vi "Create Server.vi"(5 "Server Key File (.key)":path, 7 "Server Certificate File (.crt)":path, 8 "error in (no error)":errorcluster, 11 "Server Address":string) -> (0 "error out":errorcluster, 3 "OOP Server out":refnum<class "Template Server.lvclass">)   [LabVIEW 2019, in "Template Server.lvlib" / "Template Server.lvclass"]
uses:
  Template Server.lvclass
  Template Server.lvclass/Template Server.ctl
  gRPC interface/gprc-lvsupport.lvlib
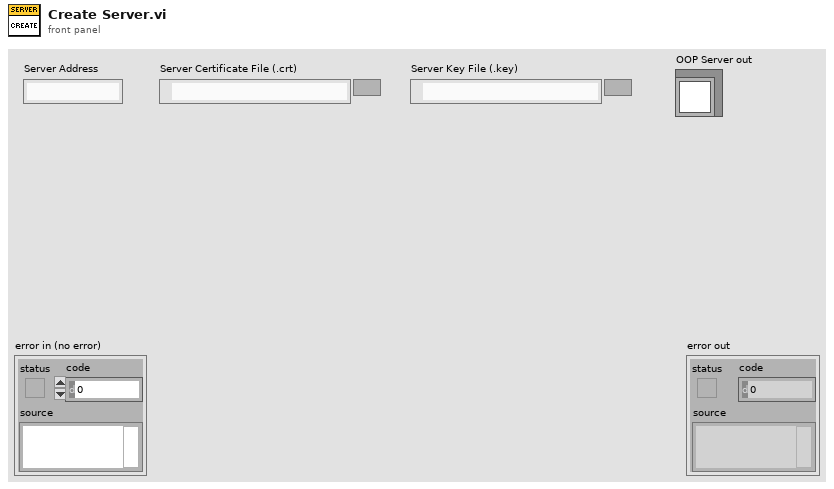
[diagram p1: front panel]
types:
  T1 = typedef "gprc-lvsupport.lvlib/grpcId.ctl" = u64
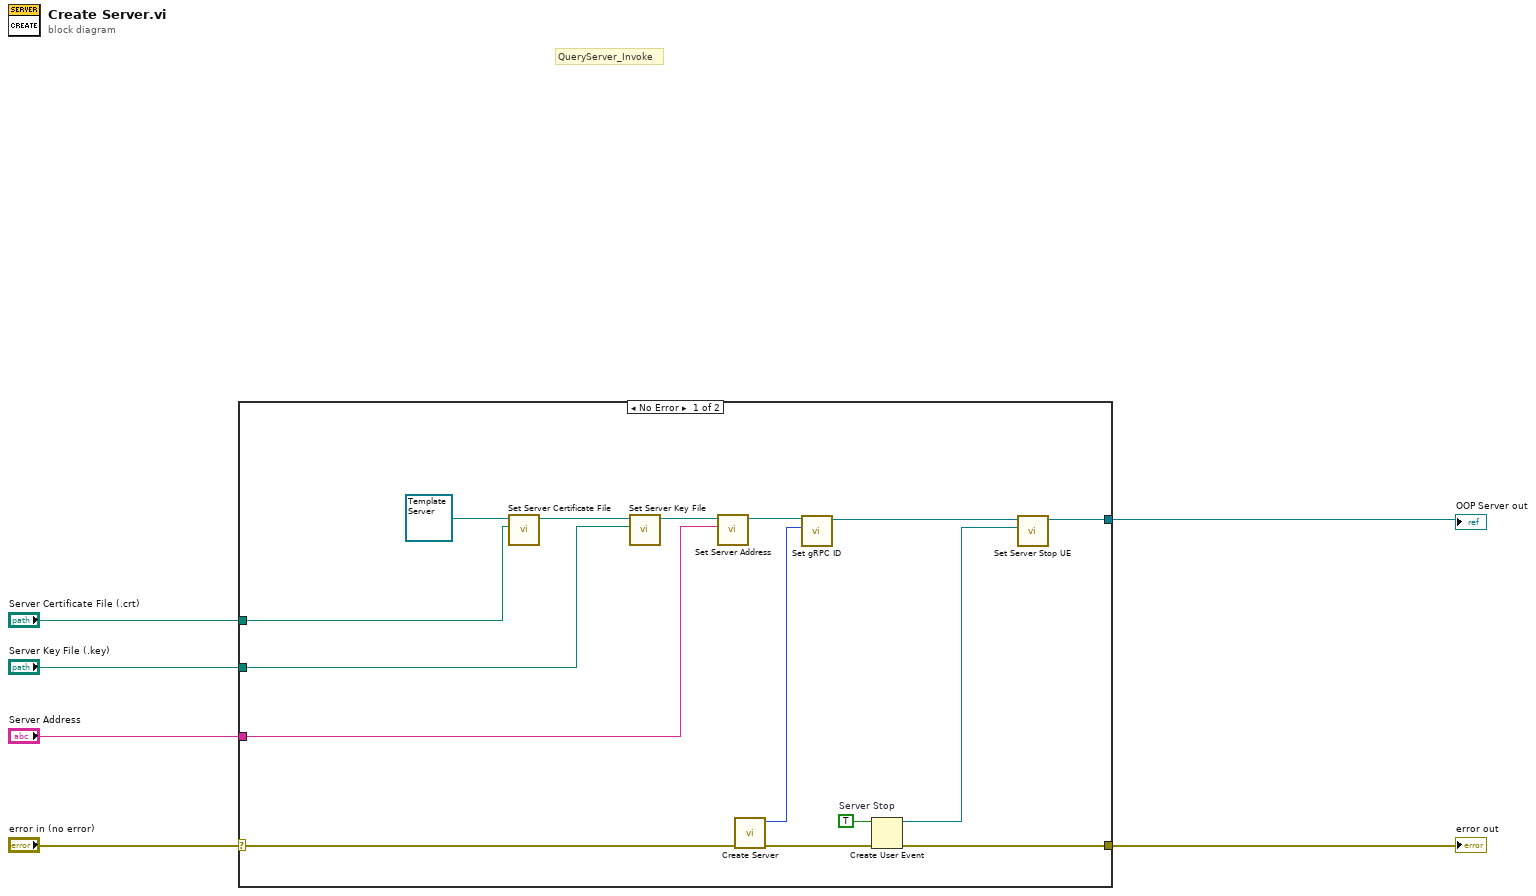
[diagram p0: block diagram]
diagram:
  # "QueryServer_Invoke"
  n1 = case shown="No Error" "error in (no error)" {
    selector: "error in (no error)" -> [w21 w22]
    tunnel: [w8 w22] -> w5
    tunnel: [w7 _] -> w4
    tunnel: "Server Certificate File (.crt)" -> [w16 _]
    tunnel: "Server Key File (.key)" -> [w15 _]
    tunnel: "Server Address" -> [w14 _]
    frame No Error {
      w12 = TRUE  # Server Stop
      n2 = call "Set Server Certificate File.vi"("Server Certificate File (.crt)"=w16, "OOP Server in"=refnum<class "Template Server.lvclass"> refnum ("OOP Server out")) -> ("OOP Server out"=w19:refnum<class "Template Server.lvclass">)  [unwired: 9 in]
      n3 = call "Set Server Key File.vi"("Server Key File (.key)"=w15, "OOP Server in"=w19) -> ("OOP Server out"=w18:refnum<class "Template Server.lvclass">)  [unwired: 9 in]
      n4 = call "Set Server Address.vi"("Server Address"=w14, "OOP Server in"=w18) -> ("OOP Server out"=w17:refnum<class "Template Server.lvclass">)  [unwired: 9 in]
      n5 = call "Create Server.vi"("error in (no error)"=w21) -> ("error out"=w10:errorcluster, "gRPCid"=w13:T1)  [unwired: 9 in]
      n6 = call "Set gRPC ID.vi"("gRPC ID"=w13, "OOP Server in"=w17) -> ("OOP Server out"=w11:refnum<class "Template Server.lvclass">)  [unwired: 9 in]
      n7 = Create User Event(user event datatype=w12, error in=w10) -> (user event=w9:refnum<user-event>, error out=w8:errorcluster)
      n8 = call "Set Server Stop UE.vi"("Server Stop UE"=w9, "OOP Server in"=w11) -> ("OOP Server out"=w7:refnum<class "Template Server.lvclass">)  [unwired: 9 in]
    }
    frame Error {
    }
  }
  "error out" <- w5
  "OOP Server out" <- w4
